vi "PathPlanner_Trajectory_WriteCSVFileIndividualState.vi"(9 "PathPlannerState":T1={"TimeSeconds"=0.0, "VelocityMPS"=0.0, "AccerationMpsSq"=0.0, "HeadingAngularVelRadPerSec"=0.0, "PositionMeters"={"X"=0.0, "Y"=0.0}, "Heading"={"VALUE"=0.0, "COS"=1.0, "SIN"=0.0}, "TargetHolonomicRotation"={"VALUE"=0.0, "COS"=1.0, "SIN"=0.0}, "CurvatureRadPerMeter"=0.0, "PathPlannerConstraints"={"MaxVelocityMps;"=0.0, "MaxAccelerationMpsSq;"=0.0, "MaxAngularVelRadPsEc;"=0.0, "MaxAngularAccRadPSecSq"=0.0, "Exists"=FALSE}, "DeltaPos"=0.0} {"TargetHolonomicRotation"."SIN" format="%13.4f"; "TargetHolonomicRotation"."COS" format="%13.4f"; "TargetHolonomicRotation"."VALUE" format="%13.4f"; "Heading"."SIN" format="%13.4f"; "Heading"."COS" format="%13.4f"; "Heading"."VALUE" format="%13.4f"; "PositionMeters"."Y" format="%14.3f"; "PositionMeters"."X" format="%14.3f"}, 10 "Comment":string, 11 "Byte Stream File in":refnum<file>) -> (3 "Byte Stream File out":refnum<file>)   [LabVIEW 2019, in "PathPlanner.lvlib"]
doc: "Internal subVI used by Util_Trajectory_WriteFile (and others). This writes one trajectory state to a file.\n\nParameters:\n - Byte stream in - file stream\n - comment - comment for this line\n - TrajectoryState - The state to write\n\nReturns: \n - Byte Stream Out - file stream"
uses:
  PathPlanner.lvlib
  TypeDef/PathPlannerTrajectoryState.ctl
  <vilib>/Rock Robotics/WPI/ThirdParty/JAS_Junk/TrajLib/TypeDef/TRANSLATION2D.ctl
  <vilib>/Rock Robotics/WPI/ThirdParty/JAS_Junk/TrajLib/TypeDef/ROTATION2D.ctl
  TypeDef/PathPlannerPathConstraints.ctl
  <vilib>/Rock Robotics/WPI/ThirdParty/JAS_Junk/TrajLib/Trajectory_Library.lvlib
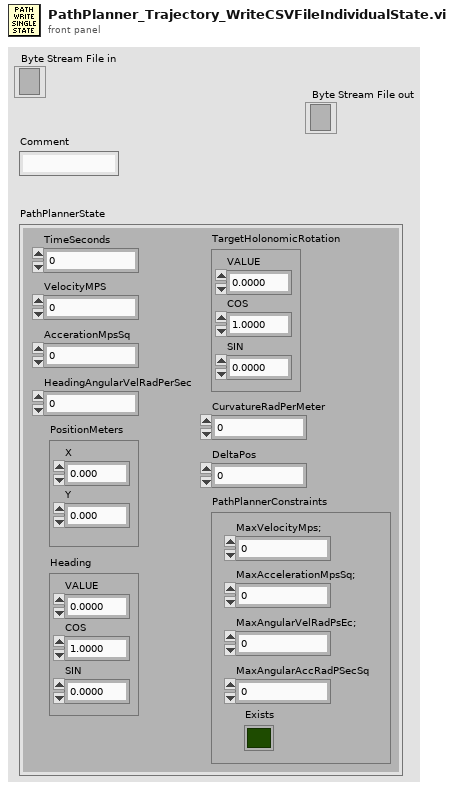
[diagram p1: front panel]
types:
  T1 = typedef "PathPlanner.lvlib/PathPlannerTrajectoryState.ctl" = cluster{"TimeSeconds":dbl, "VelocityMPS":dbl, "AccerationMpsSq":dbl, "HeadingAngularVelRadPerSec":dbl, "PositionMeters":T2, "Heading":T3, "TargetHolonomicRotation":T3, "CurvatureRadPerMeter":dbl, "PathPlannerConstraints":T4, "DeltaPos":dbl}
  T2 = typedef "Trajectory_Library.lvlib/TRANSLATION2D.ctl" = cluster{"X":dbl, "Y":dbl}
  T3 = typedef "Trajectory_Library.lvlib/ROTATION2D.ctl" = cluster{"VALUE":dbl, "COS":dbl, "SIN":dbl}
  T4 = typedef "PathPlanner.lvlib/PathPlannerPathConstraints.ctl" = cluster{"MaxVelocityMps;":dbl, "MaxAccelerationMpsSq;":dbl, "MaxAngularVelRadPsEc;":dbl, "MaxAngularAccRadPSecSq":dbl, "Exists":bool}
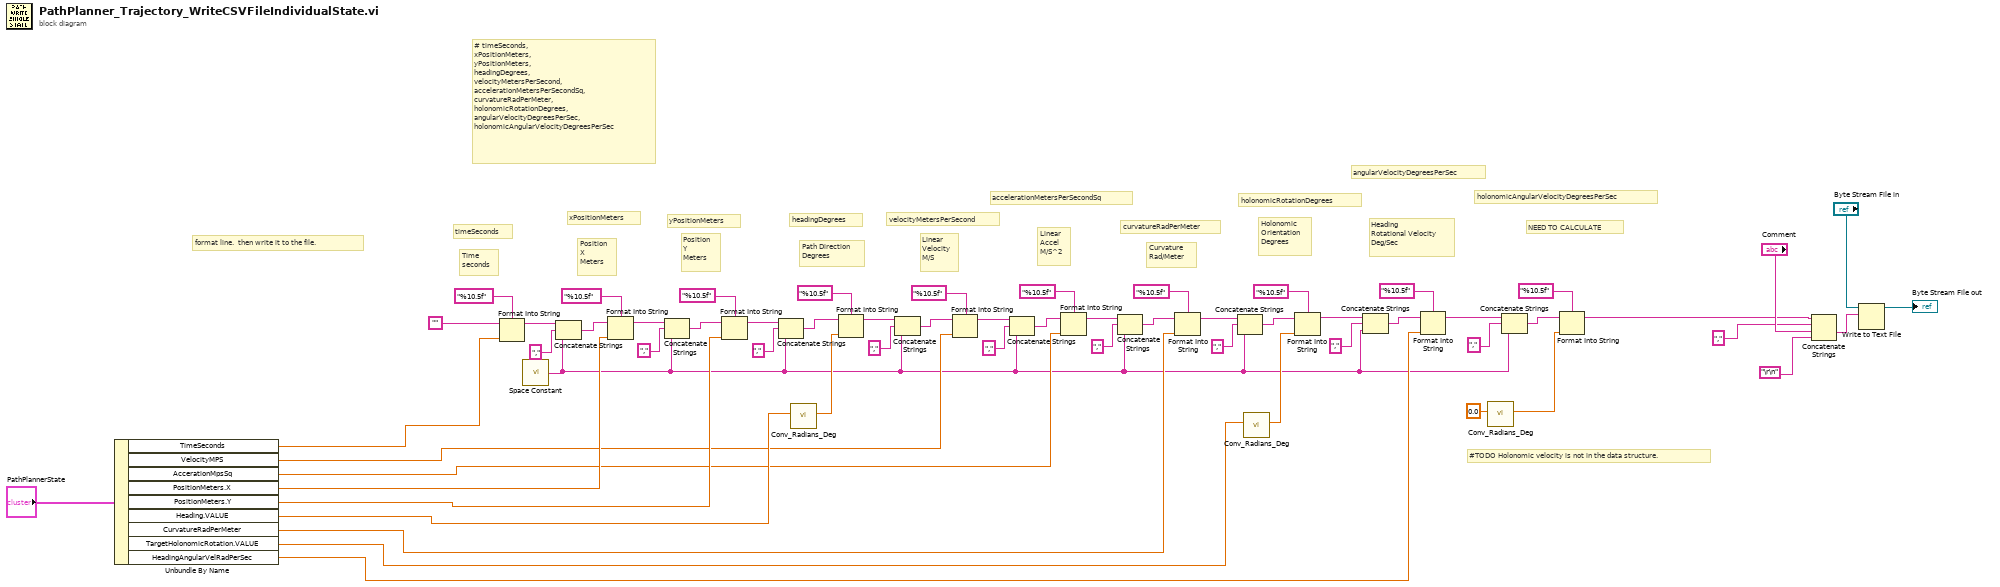
[diagram p0: block diagram]
diagram:
  # "# timeSeconds, \nxPositionMeters, \nyPositionMeters, \nheadingDegrees, \nvelocityMetersPerSecond, \naccelerationMetersPerSecondSq, \ncurvatureRadPerMeter, \nholonomicRotationDegrees, \nangularVelocityDegreesPerSec, \nholonomicAngularVelocityDegreesPerSec"
  # "NEED TO CALCULATE"
  # "#TODO Holonomic velocity is not in the data structure."
  # "holonomicAngularVelocityDegreesPerSec"
  # "angularVelocityDegreesPerSec"
  # "holonomicRotationDegrees"
  # "curvatureRadPerMeter"
  # "accelerationMetersPerSecondSq"
  # "velocityMetersPerSecond"
  # "headingDegrees"
  # "yPositionMeters"
  # "xPositionMeters"
  # "timeSeconds"
  # "Heading\nRotational Velocity\nDeg/Sec"
  # "Holonomic\nOrientation\nDegrees"
  # "Curvature\nRad/Meter"
  # "Path Direction\nDegrees"
  # "Position\nY\nMeters"
  # "Position\nX\nMeters"
  # "Linear\nAccel\nM/S^2"
  # "Linear\nVelocity\nM/S"
  # "Time\nseconds"
  # "format line.  then write it to the file."
  n1 = Unbundle By Name("PathPlannerState") -> ("TimeSeconds"=w27:dbl, "VelocityMPS"=w12:dbl, "AccerationMpsSq"=w11:dbl, "PositionMeters.X"=w16:dbl, "PositionMeters.Y"=w15:dbl, "Heading.VALUE"=w14:dbl, "CurvatureRadPerMeter"=w26:dbl, "TargetHolonomicRotation.VALUE"=w4:dbl, "HeadingAngularVelRadPerSec"=w17:dbl)
  n2 = Format Into String(format string="%10.5f", initial string="", w27) -> (resulting string=w31:string)  [unwired: 1 in, 1 out]
  n3 = call <vilib>:"Space Constant.vi"() -> ("String"=w2:string)
  n4 = Concatenate Strings(w31, "," ("string"), w2) -> (w41:string)
  n5 = Format Into String(format string="%10.5f", initial string=w41, w16) -> (resulting string=w34:string)  [unwired: 1 in, 1 out]
  n6 = Concatenate Strings(w34, "," ("string"), w2) -> (w40:string)
  n7 = Format Into String(format string="%10.5f", initial string=w40, w15) -> (resulting string=w37:string)  [unwired: 1 in, 1 out]
  n8 = Concatenate Strings(w37, "," ("string"), w2) -> (w55:string)
  n9 = call <vilib>:"Conv_Radians_Deg.vi"("Radians"=w14) -> ("Degrees"=w13:dbl)  [unwired: 10 in]
  n10 = Format Into String(format string="%10.5f", initial string=w55, w13) -> (resulting string=w42:string)  [unwired: 1 in, 1 out]
  n11 = Concatenate Strings(w42, "," ("string"), w2) -> (w48:string)
  n12 = Format Into String(format string="%10.5f", initial string=w48, w12) -> (resulting string=w45:string)  [unwired: 1 in, 1 out]
  n13 = Concatenate Strings(w45, "," ("string"), w2) -> (w54:string)
  n14 = Format Into String(format string="%10.5f", initial string=w54, w11) -> (resulting string=w49:string)  [unwired: 1 in, 1 out]
  n15 = Concatenate Strings(w49, "," ("string"), w2) -> (w53:string)
  n16 = Format Into String(format string="%10.5f", initial string=w53, w26) -> (resulting string=w19:string)  [unwired: 1 in, 1 out]
  n17 = Concatenate Strings(w19, "," ("string"), w2) -> (w25:string)
  n18 = call <vilib>:"Conv_Radians_Deg.vi"("Radians"=w4) -> ("Degrees"=w10:dbl)  [unwired: 10 in]
  n19 = Format Into String(format string="%10.5f", initial string=w25, w10) -> (resulting string=w18:string)  [unwired: 1 in, 1 out]
  n20 = Concatenate Strings(w18, "," ("string"), w2) -> (w22:string)
  n21 = Format Into String(format string="%10.5f", initial string=w22, w17) -> (resulting string=w6:string)  [unwired: 1 in, 1 out]
  n22 = call <vilib>:"Conv_Radians_Deg.vi"("Radians"=0.0) -> ("Degrees"=w3:dbl)  [unwired: 10 in]
  n23 = Concatenate Strings(w6, "," ("string"), w2) -> (w9:string)
  n24 = Format Into String(format string="%10.5f", initial string=w9, w3) -> (resulting string=w5:string)  [unwired: 1 in, 1 out]
  n25 = Concatenate Strings(w5, "," ("string"), "Comment", "\r\n") -> (w57:string)
  n26 = Write to Text File(file (use dialog)="Byte Stream File in", text=w57) -> (refnum out=→"Byte Stream File out":refnum<file>)  [unwired: 2 in, 2 out]
